vi "Create New Test Executive.vi"(8 "error in (no error)":errorcluster, 10 "Name":string, 11 "Test Executive":refnum<class "ITest Executive.lvclass">) -> (0 "error out":errorcluster, 3 "Test Executive Ref":refnum<data-value>, 5 "Test Executive ID out":string)   [LabVIEW 2020, in "Test Executive.lvlib" / "TestExecutive Ref.lvclass"]
uses:
  <vilib>/gpm_packages/@cs/test-executive/Source/Test Executive/TestExecutive Ref/TestExecutive Ref.lvclass
  <vilib>/gpm_packages/@cs/test-executive/Source/Test Executive/ITestExecutive/ITest Executive.lvclass
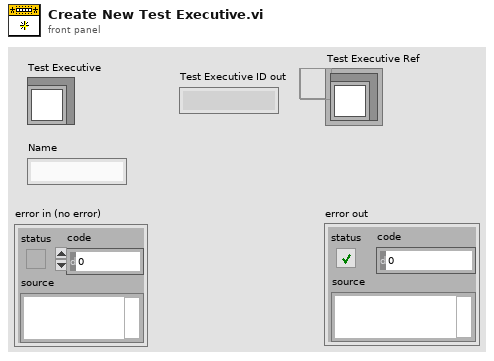
[diagram p1: front panel]
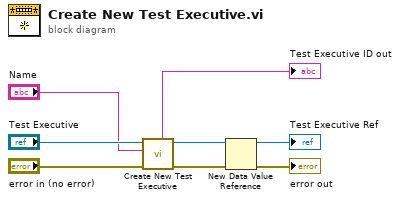
[diagram p0: block diagram]
diagram:
  n1 = call-dynamic "Create New Test Executive.vi"("error in (no error)"="error in (no error)", "Name"="Name", "ITest Executive in"="Test Executive") -> ("error out"=w3:errorcluster, "ITest Executive out"=w4:refnum<class "ITest Executive.lvclass">, "Unique ID out"=→"Test Executive ID out":string)  [unwired: 6 in]
  n2 = New Data Value Reference(data value=w4, error in=w3) -> (data value reference=→"Test Executive Ref":refnum<data-value>, error out=→"error out":errorcluster)
